vi "Update Waveform List.vi"(8 "error in (no error)":errorcluster, 10 "Waveform Listbox Ref":refnum<vi>, 11 "Data In":T1 {"Toggle Channels"."Initial State" items=["High"=101, "Low"=102]; "Sample Rate" format="%.2p"}) -> (0 "error out":errorcluster, 3 "Data Out":T1 {"Toggle Channels"."Initial State" items=["High"=101, "Low"=102]; "Sample Rate" format="%.2p"})   [LabVIEW 2021]
uses:
  <vilib>/express/express signal manip/GetorSetDDTAttributes/Get DDT Attributes/Get DDT Properties.xnode
  <vilib>/express/express shared/transition.llb/Dynamic To Waveform Array.vi
  <vilib>/express/express signal manip/GetorSetDDTAttributes/Set DDT Attributes/Set DDT Properties.xnode
  <vilib>/express/express signal manip/GetorSetDDTAttributes/Set DDT Attributes/SetT0.vi
  <vilib>/express/express shared/transition.llb/Waveform Array To Dynamic.vi
  Controls/Script Trigger Routing.ctl
  Controls/Toggle Channel.ctl
  Controls/Data.ctl
panel:
  out "Table":string[][](array[string])
  out "Duration (s)":dbl[](array[numeric]) format="%#_6p"
  out "Size":i32[](array[numeric])
  out "Wfm Names":string[](array[string])
  # "#Debug Use"
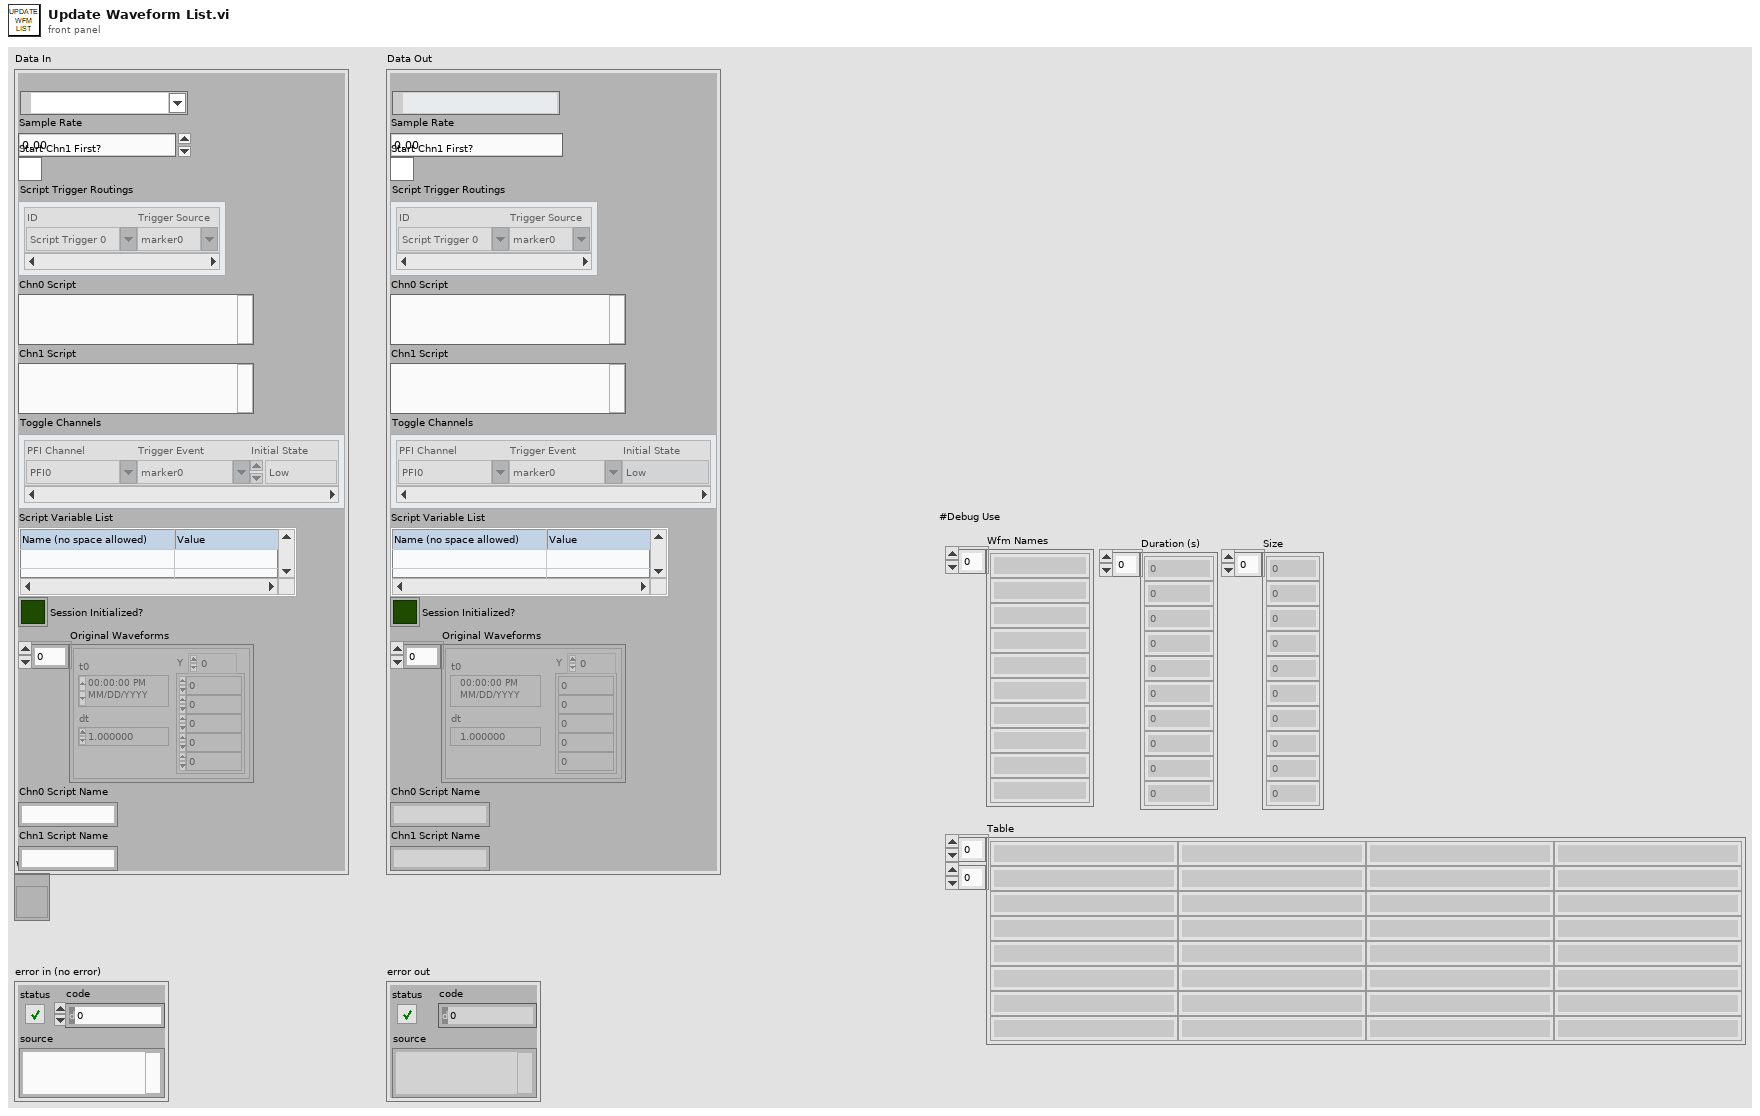
[diagram p1: front panel]
types:
  T1 = typedef "Data.ctl" = cluster{"FGEN Resource Name":refnum<k15>, "Sample Rate":dbl, "Start Chn1 First?":bool, "Script Trigger Routings":T2[], "Chn0 Script":string, "Chn1 Script":string, "Toggle Channels":T3[], "Script Variable List":string[][], "Session Initialized?":bool, "Original Waveforms":waveform(dbl)[], "Chn0 Script Name":string, "Chn1 Script Name":string}
  T2 = typedef "Script Trigger Routing.ctl" = cluster{"ID":string, "Trigger Source":string}
  T3 = typedef "Toggle Channel.ctl" = cluster{"PFI Channel":string, "Trigger Event":string, "Initial State":u16}
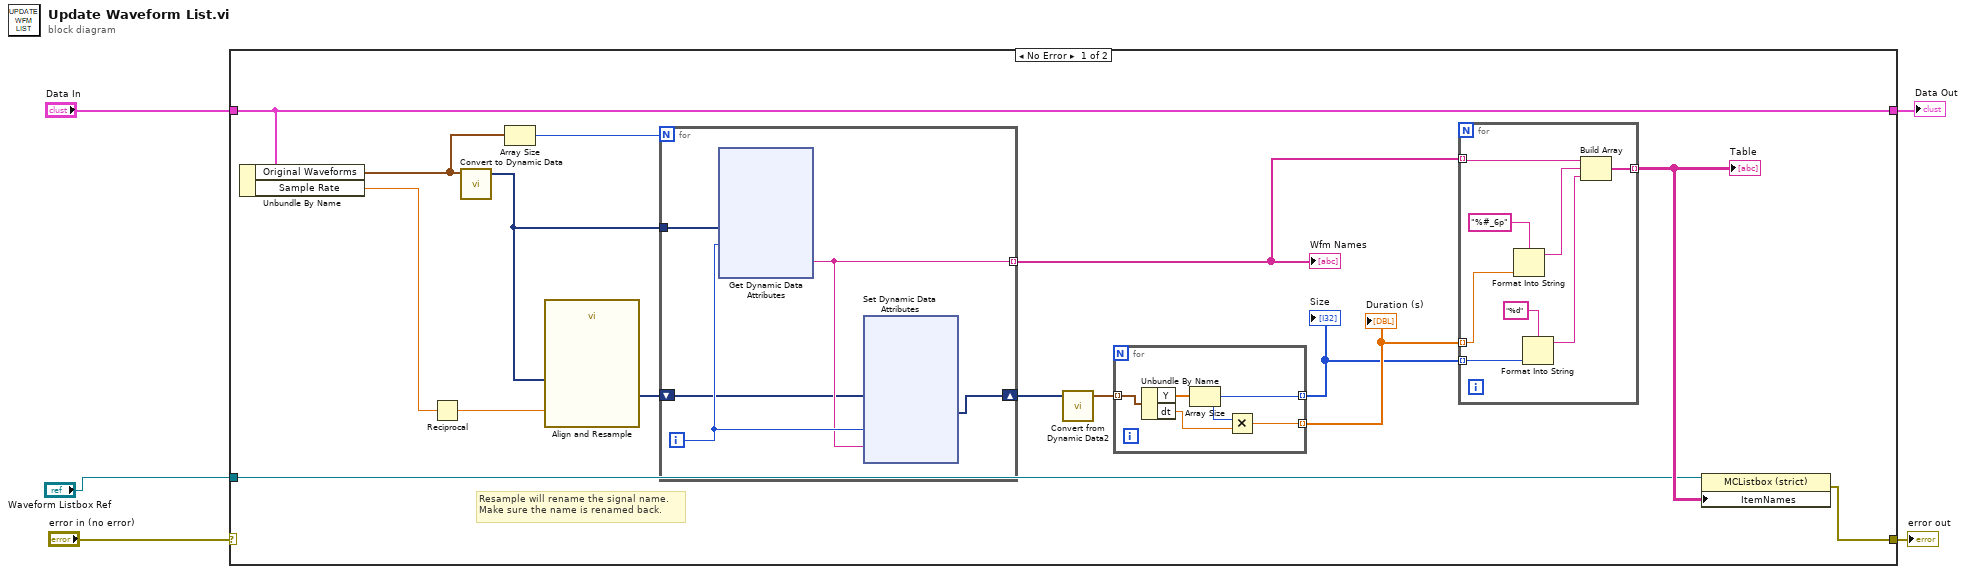
[diagram p0: block diagram]
diagram:
  n1 = case shown="No Error" "error in (no error)" {
    selector: "error in (no error)" -> [_ w62]
    tunnel: "Data In" -> [w20 w61]
    tunnel: [w20 w61] -> w4
    tunnel: [w13 w62] -> w2
    tunnel: "Waveform Listbox Ref" -> [w9 _]
    frame No Error {
      # "Resample will rename the signal name.\nMake sure the name is renamed back."
      n2 = Unbundle By Name(w20) -> ("Original Waveforms"=w16:waveform(dbl)[], "Sample Rate"=w19:dbl)
      n3 = Reciprocal(x=w19) -> (1/x=w18:dbl)
      n4 = call "Convert to Dynamic Data"("Array of Waveforms"=w16) -> ("Dynamic Data Type"=w6:dynamicdata)  [unwired: 3 in]
      n5 = Array Size(array=w16) -> (size(s)=w15:i32)
      n6 = call "Align and Resample"("dt"=w18, "Signals"=w6) -> ("Resampled Signals"=w8:dynamicdata)  [unwired: 7 in, 2 out]
      n7 = for {
        N: w15 -> [_]
        tunnel: [w37] -> w14 mode=indexing
        shift-right: [w36] -> w7
        shift-left: w8 -> [w35]
        tunnel: w6 -> [w34]
        i -> [w38]
        n8 = xnode "Get Dynamic Data Attributes"("Signals In"=w34, "Signal Index"=w38) -> ("Signal Name"=w37:string)  [unwired: 1 in, 2 out]
        n9 = xnode "Set Dynamic Data Attributes"("Signals In"=w35, "Signal Index"=w38, "Signal Name"=w37) -> ("Signals Out"=w36:dynamicdata)  [unwired: 1 in, 1 out]
      }
      "Wfm Names" <- w14
      n10 = call "Convert from Dynamic Data2"("Dynamic Data Type"=w7) -> ("Array of Waveform"=w17:waveform(dbl)[])  [unwired: 3 in]
      n11 = for {
        tunnel: w17 -> [w33] mode=indexing
        tunnel: [w31] -> w11 mode=indexing
        tunnel: [w30] -> w10 mode=indexing
        n12 = Unbundle By Name(w33) -> ("Y"=w32:dbl[], "dt"=w29:dbl)
        n13 = Array Size(array=w32) -> (size(s)=w30:i32)
        n14 = Multiply(x=w30, y=w29) -> (x*y=w31:dbl)
      }
      "Size" <- w10
      "Duration (s)" <- w11
      n15 = for {
        tunnel: w14 -> [w24] mode=indexing
        tunnel: w11 -> [w27] mode=indexing
        tunnel: w10 -> [w25] mode=indexing
        tunnel: [w21] -> w12 mode=indexing
        n16 = Format Into String(format string="%#_6p", w27) -> (resulting string=w23:string)  [unwired: 2 in, 1 out]
        n17 = Format Into String(format string="%d", w25) -> (resulting string=w22:string)  [unwired: 2 in, 1 out]
        n18 = Build Array(w24, w23, w22) -> (w21:string[])
      }
      "Table" <- w12
      n19 = property class="MCListbox (strict)"(reference=w9, "ItemNames"=w12) -> (error out=w13:errorcluster)  [unwired: 1 in, 1 out]
    }
    frame Error {
    }
  }
  "Data Out" <- w4
  "error out" <- w2
